vi "SetParam.vi"(8 "error in (no error)":errorcluster caption="entrée d'erreur (pas d'erreur)", 10 "OrdinalEncoder":cluster{"dtype":string}={"dtype"="float"}, 11 "OrdinalEncoder.lvclass":refnum<class "OrdinalEncoder.lvclass">) -> (0 "error out":errorcluster caption="sortie d'erreur", 3 "OrdinalEncoder.lvclass":refnum<class "OrdinalEncoder.lvclass">)   [LabVIEW 2020, in "OrdinalEncoder.lvclass"]
doc: "Set Parameters"
uses:
  OrdinalEncoder.lvclass
  OrdinalEncoder.lvclass/OrdinalEncoder.ctl
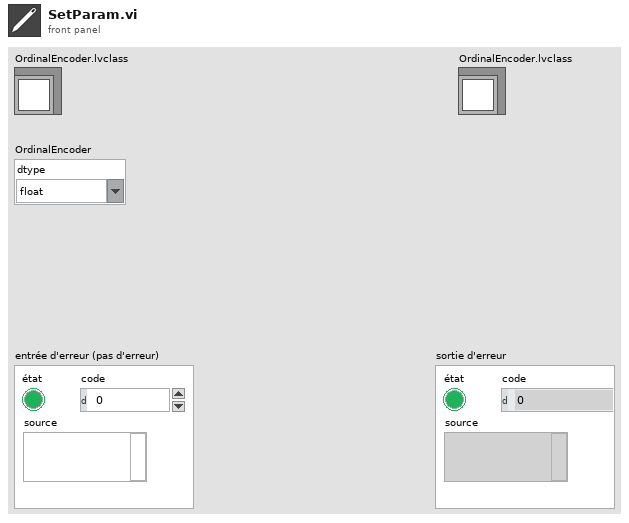
[diagram p1: front panel]
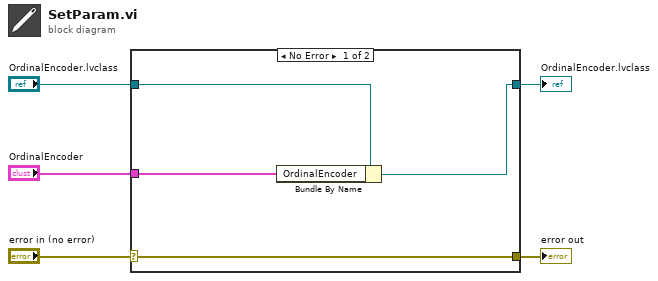
[diagram p0: block diagram]
diagram:
  n1 = case shown="No Error" "error in (no error)" {
    selector: "error in (no error)" -> [w9 w10]
    tunnel: [w9 w10] -> w4
    tunnel: [w7 w11] -> w2
    tunnel: "OrdinalEncoder.lvclass" -> [w8 w11]
    tunnel: "OrdinalEncoder" -> [w6 _]
    frame No Error {
      n2 = Bundle By Name(cluster=w8, "OrdinalEncoder"=w6) -> (w7:refnum<class "OrdinalEncoder.lvclass">)
    }
    frame Error {
    }
  }
  "error out" <- w4
  "OrdinalEncoder.lvclass" <- w2
